vi "FlatToRichstreamtest_Empty.vi"(5 "OutputClusterType":T1, 11 "InputCluster":T2) -> (3 "OutputCluster":T1)   [LabVIEW 2021, in "streamtest_client.lvlib"]
uses:
  streamtest_client.lvlib
  streamtest_Empty_Flat.ctl
  streamtest_Empty.ctl
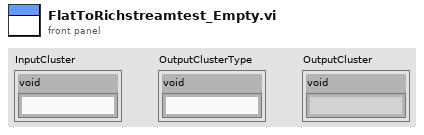
[diagram p1: front panel]
types:
  T1 = typedef "streamtest_client.lvlib/streamtest_Empty.ctl" = cluster{"void":string}
  T2 = typedef "streamtest_client.lvlib/streamtest_Empty_Flat.ctl" = cluster{"void":string}
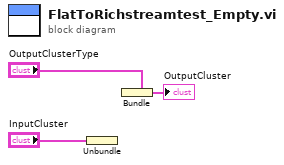
[diagram p0: block diagram]
diagram:
  n1 = Unbundle "Unbundle"("InputCluster") -> ()  [unwired: 1 out]
  n2 = Bundle "Bundle"(cluster="OutputClusterType") -> (→"OutputCluster":T1)  [unwired: 1 in]
